vi "Main.vi"() -> ()   [LabVIEW 2021]
uses:
  <vilib>/Instr/_visa.llb/VISA Configure Serial Port (Instr).vi
panel:
  out "Waveform Chart":cluster{"ADC":u32, "Timestamp":u32}(graph)
  out "remaining string":string
  out "error out":errorcluster
  in  "stop":bool
  in  "VISA resource name":refnum<visa-resource-name>
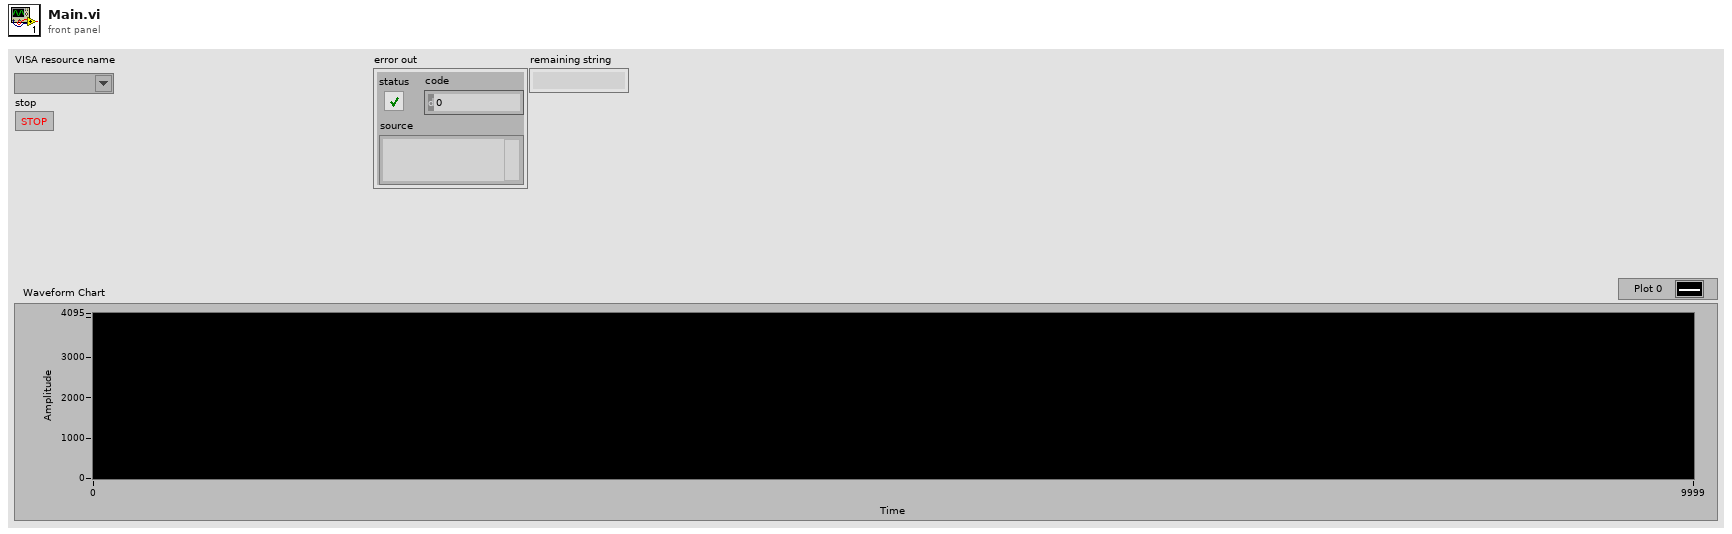
[diagram p1: front panel]
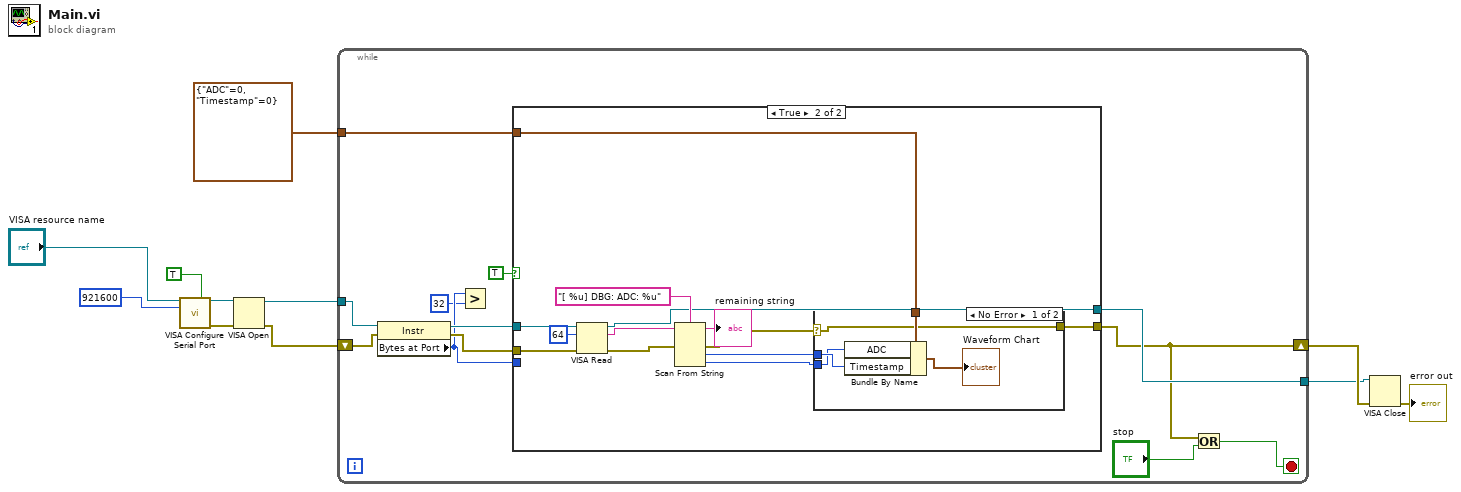
[diagram p0: block diagram]
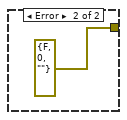
[diagram p3: hidden frame]
diagram:
  n1 = call-poly "VISA Configure Serial Port"("VISA resource name"="VISA resource name", "Enable Termination\nChar (T)"=TRUE ("Enable Termination\nChar (T)"), "baud rate (9600)"=u32 921600) -> ("VISA resource name out"=w7:refnum<visa-resource-name>, "error out"=w8:errorcluster)  [unwired: 11 in]
  n2 = VISA Open(error in (no error)=w8, VISA resource name=w7) -> (VISA resource name=w6:refnum<visa-resource-name>, error out=w5:errorcluster)  [unwired: 3 in]
  n3 = while {
    tunnel: w6 -> [w23]
    tunnel: cluster{"ADC":u32, "Timestamp":u32} {"ADC"=0, "Timestamp"=0} -> [w19]
    shift-right: [w12] -> w3
    shift-left: w5 -> [w20]
    tunnel: [w18] -> w2
    stop <- w13 stop-if-true
    n4 = property class="Instr"(reference=w23, error in=w20) -> (reference out=w22:refnum<visa-resource-name>, error out=w21:errorcluster, "Bytes at Port"=w17:u32)
    n5 = Greater?(x=w17, y=u32 32) -> ()  [unwired: 1 out]
    n6 = case shown="True" TRUE {
      tunnel: w22 -> [w24 w38]
      tunnel: w21 -> [w25 w37]
      tunnel: w19 -> [_ w33]
      tunnel: [w25 w30] -> w12
      tunnel: [w24 w32] -> w18
      tunnel: w17 -> [_ _]
      frame False {
      }
      frame True {
        n7 = VISA Read(VISA resource name=w38, byte count=u32 64, error in (no error)=w37) -> (VISA resource name out=w32:refnum<visa-resource-name>, read buffer=w35:string, error out=w36:errorcluster)  [unwired: 1 out]
        n8 = Scan From String(format string="[ %u] DBG: ADC: %u", input string=w35, error in=w36) -> (remaining string=→"remaining string":string, error out=w29:errorcluster, output 1=w28:u32, output 2=w27:u32)  [unwired: 3 in, 1 out]
        n9 = case shown="No Error" w29 {
          selector: w29 -> [w42 _]
          tunnel: w33 -> [w43 _]
          tunnel: [w42 errorcluster {"status"=FALSE, "code"=0, "source"=""} ("error out")] -> w30
          tunnel: w28 -> [w41 _]
          tunnel: w27 -> [w40 _]
          frame No Error {
            n10 = Bundle By Name(cluster=w43, "ADC"=w40, "Timestamp"=w41) -> (→"Waveform Chart":cluster{"ADC":u32, "Timestamp":u32})
          }
          frame Error {
          }
        }
      }
    }
    n11 = Or(x=w12, y="stop") -> (x .or. y?=w13:bool)
  }
  n12 = VISA Close(VISA resource name=w2, error in (no error)=w3) -> (error out=→"error out":errorcluster)
